vi "Route Pin To String.vi"(10 "Pin":T1, 11 "Module":string) -> (2 "String":string)   [LabVIEW 2017, in "Chassis TimeSync Engine.lvlib"]
uses:
  Chassis TimeSync Engine.lvlib
  Timekeeper Route Pin.ctl
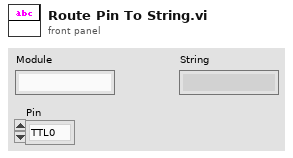
[diagram p1: front panel]
types:
  T1 = typedef "Chassis TimeSync Engine.lvlib/Timekeeper Route Pin.ctl" = enum16{"TTL0", "TTL1", "PFI0", "PFI1", "PFI2", "PXI_Clk10", "PXI_Clk10_In", "BoardClk", "ClkOut", "Oscillator"}
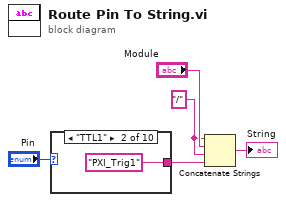
[diagram p0: block diagram]
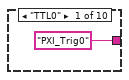
[diagram p2: hidden frame]
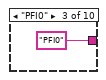
[diagram p3: hidden frame]
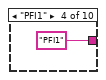
[diagram p4: hidden frame]
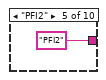
[diagram p5: hidden frame]
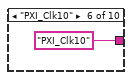
[diagram p6: hidden frame]
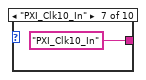
[diagram p7: hidden frame]
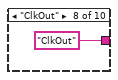
[diagram p8: hidden frame]
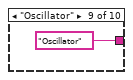
[diagram p9: hidden frame]
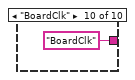
[diagram p10: hidden frame]
diagram:
  w4 = "/" ("string")
  n1 = case shown="\"TTL1\"" "Pin" {
    tunnel: ["PXI_Trig0" ("string") "PXI_Trig1" ("string") "PFI0" ("string") "PFI1" ("string") "PFI2" ("string") "PXI_Clk10" ("string") "PXI_Clk10_In" ("string") "ClkOut" ("string") "Oscillator" ("string") "BoardClk" ("string")] -> w2
    frame "TTL0" {
    }
    frame "TTL1" {
    }
    frame "PFI0" {
    }
    frame "PFI1" {
    }
    frame "PFI2" {
    }
    frame "PXI_Clk10" {
    }
    frame "PXI_Clk10_In" {
    }
    frame "ClkOut" {
    }
    frame "Oscillator" {
    }
    frame "BoardClk" {
    }
  }
  n2 = Concatenate Strings(w4, "Module", w4, w2) -> (→"String":string)
